vi "Power Off.vi"(8 "error in (no error)":errorcluster, 11 "VISA resource name":refnum<visa-resource-name>) -> (0 "error out":errorcluster, 3 "VISA resource name out":refnum<visa-resource-name>)   [LabVIEW 2015, in "Ohaus AV Series.lvlib"]
doc: "This VI switches balance's power off."
uses:
  <instrlib>/Ohaus AV Series/Ohaus AV Series.lvlib
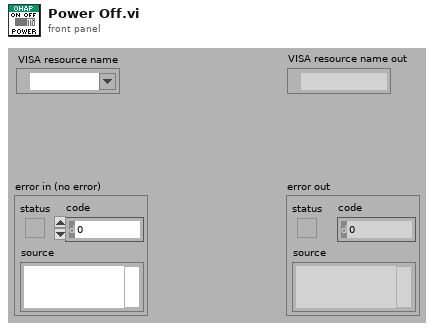
[diagram p1: front panel]
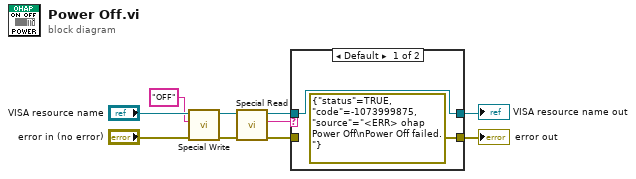
[diagram p0: block diagram]
diagram:
  n1 = call <instrlib>:"Special Write.vi"("error in (no error)"="error in (no error)", "Input String"="OFF", "VISA resource name"="VISA resource name") -> ("error out"=w9:errorcluster, "VISA resource name out"=w4:refnum<visa-resource-name>)  [unwired: 7 in]
  n2 = call <instrlib>:"Special Read.vi"("error in (no error)"=w9, "VISA resource name"=w4) -> ("error out"=w6:errorcluster, "Output String"=w3:string, "VISA resource name out"=w5:refnum<visa-resource-name>)  [unwired: 7 in]
  n3 = case shown="Default" w3 {
    tunnel: [errorcluster {"status"=TRUE, "code"=-1073999875, "source"="<ERR> ohap Power Off\nPower Off failed."} ("error out") w14] -> w10
    tunnel: w5 -> [w11 w13]
    tunnel: w6 -> [_ w14]
    tunnel: [w11 w13] -> w1
    frame Default {
    }
    frame "OK!\r\n" {
    }
  }
  "error out" <- w10
  "VISA resource name out" <- w1
